vi "ProdaNG.TestValueResult.New.vi"(8 "error in (no error)":errorcluster, 10 "TestValueResult":T1, 11 "dbHandle":i32) -> (0 "error out":errorcluster, 3 "dbHandle":i32)   [LabVIEW 2016]
doc: "This function changes the process step result, which is defined by a ProcessStepResult structure. A process step result can either be set intentionally or leave the check of the test step results and the resulting changes to the DLL. In case, that the DLL changes the Process Result, the mdTime of the according Product is set to the current time and the mdProcessStepId is set to this process step. \nThe automatic check stands to the following rule:\n1. It is checked, if all test steps have the Status IO.\nIf the result of the test is IO, the status 1 (IO) is set in the test value result, otherwise the status 0 (NIO), respective 5 (IO Repeat) or 6 (NIO Repeat) in case of a repeat.\nParameter:\nhandle is an Integer, which is returned by the function Login() at the creation of a new connection.\nisRepeat shows, if this step is a repeat.\nprocessStepResult is a pointer on a ProcessStepResult structure, which elements must be prefilled. The structure must be defined and filled in the calling program. Changes can only be made on the elements StatusId, startTime and endTime. If the Endtime is not set, it is automatically filled with the current time by the DLL. \nThe element statusId is of particular importance:\nIf this element is passed with the value -1, the DLL makes a check on the test step results and sets the changeable elements automatically. Otherwise the returned values for status, start time and end time are set.\n\nReturncodes:\n0 No error\n< 0 ORACLE Error code\n6 (ERROR_INVALID_HANDLE) in case of an invalid handle\n1403 Record does not exist"
uses:
  Controls/ProdaNG.TestValueResult.ctl
  Controls/ProdaNG.TestValueResultSize.ctl
  prodllNG.dll
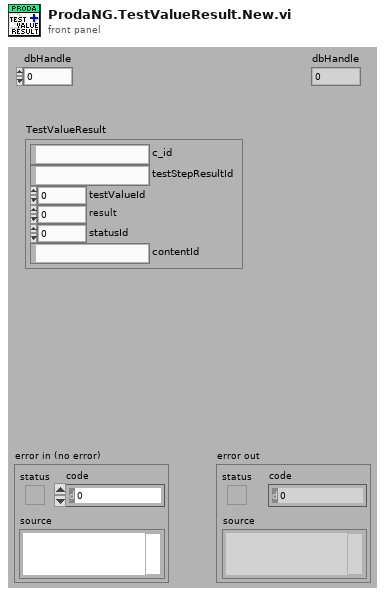
[diagram p1: front panel]
types:
  T1 = typedef "ProdaNG.TestValueResult.ctl" = cluster{"c_id":string, "testStepResultId":string, "testValueId":i32, "result":dbl, "statusId":i32, "contentId":string}
  T2 = typedef "ProdaNG.TestValueResultSize.ctl" = cluster{"c_id":i32, "testStepResultId":i32, "testValueId":i32, "result":i32, "statusId":i32, "contentId":i32}
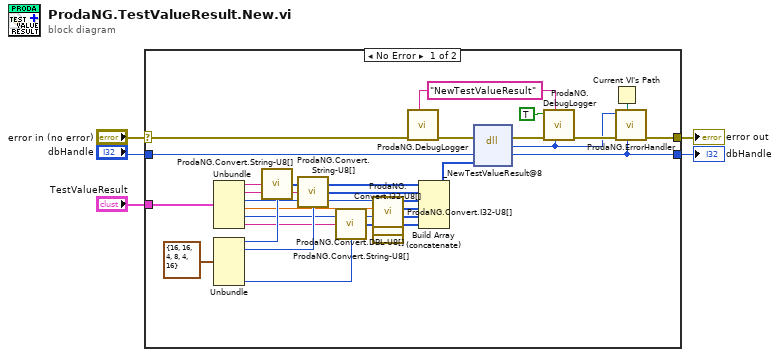
[diagram p0: block diagram]
diagram:
  n1 = case shown="No Error" "error in (no error)" {
    selector: "error in (no error)" -> [w16 w36]
    tunnel: [w13 w36] -> w4
    tunnel: [w12 w35] -> w3
    tunnel: "dbHandle" -> [w15 w35]
    tunnel: "TestValueResult" -> [w14 _]
    frame No Error {
      w31 = "NewTestValueResult" ("cmd")
      n2 = Unbundle(w14) -> ("c_id"=w33:string, "testStepResultId"=w34:string, "testValueId"=w21:i32, "result"=w20:dbl, "statusId"=w10:i32, "contentId"=w9:string)
      n3 = Unbundle(T2 {"c_id"=16, "testStepResultId"=16, "testValueId"=4, "result"=8, "statusId"=4, "contentId"=16} ("TestValueResultSize")) -> ("c_id"=w25:i32, "testStepResultId"=w23:i32, "contentId"=w6:i32)  [unwired: 3 out]
      n4 = call "ProdaNG.Convert.String-U8[].vi"("Input String"=w33, "Size"=w25) -> ("Output"=w24:u8[])
      n5 = call "ProdaNG.Convert.String-U8[].vi"("Input String"=w34, "Size"=w23) -> ("Output"=w22:u8[])
      n6 = call "ProdaNG.Convert.String-U8[].vi"("Input String"=w9, "Size"=w6) -> ("Output"=w8:u8[])
      n7 = call "ProdaNG.Convert.I32-U8[].vi"("32bit integer"=w21) -> ("unsigned byte array"=w19:u8[])  [unwired: 10 in]
      n8 = call "ProdaNG.Convert.DBL-U8[].vi"("dbl"=w20) -> ("unsigned byte array"=w18:u8[])  [unwired: 10 in]
      n9 = call "ProdaNG.Convert.I32-U8[].vi"("32bit integer"=w10) -> ("unsigned byte array"=w11:u8[])  [unwired: 10 in]
      n10 = call "ProdaNG.DebugLogger.vi"("cmd"=w31, "error in (no error)"=w16) -> ("error out"=w26:errorcluster)  [unwired: 9 in]
      n11 = Build Array (concatenate)(w24, w22, w19, w18, w11, w8) -> (w17:u8[])
      n12 = dll-call lib="D:/Maszup/WABCO/SVN/LineTraceSystem/SOFTWARE/sources/Database/ProdaNG/prodllNG.dll" fn="_NewTestValueResult@8" ("ProDll.dll:InitProDll")(error in=w26, "dbHandle"=w15, "testValueResult"=w17) -> (error out=w29:errorcluster, "return type"=w27:i32, "dbHandle"=w12:i32)  [unwired: 3 in, 1 out]
      n13 = call "ProdaNG.DebugLogger.vi"("return type"=w27, "cmd"=w31, "error in (no error)"=w29, "done? (F)"=TRUE) -> ("error out"=w28:errorcluster)  [unwired: 7 in]
      n14 = Current VI's Path() -> (path=w32:path)
      n15 = call "ProdaNG.ErrorHandler.vi"("dbHandleIn"=w12, "Path"=w32, "error in"=w28, "output_parameter"=w27) -> ("error out"=w13:errorcluster)  [unwired: 7 in]
    }
    frame Error {
    }
  }
  "error out" <- w4
  "dbHandle" <- w3
